vi "GetAllQueues.vi"(8 "error in (no error)":errorcluster, 11 "Qbus in":refnum<class "Qbus.lvclass">) -> (0 "error in (no error)":errorcluster, 2 "queues":refnum<queue>[](array[refnum]), 3 "Qbus out":refnum<class "Qbus.lvclass">)   [LabVIEW 2017, in "Qbus.lvclass"]
uses:
  <vilib>/addons/Qbus/Qbus.lvclass
  <vilib>/addons/Qbus/controls/message.ctl
  <vilib>/addons/Qbus/Qbus.lvclass/Qbus.ctl
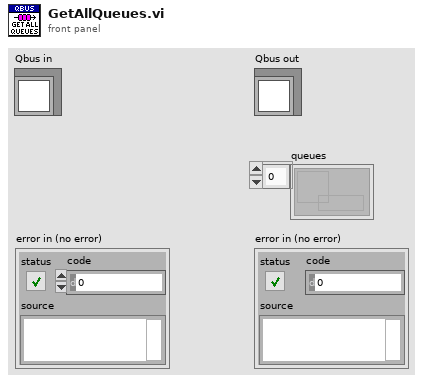
[diagram p1: front panel]
types:
  T1 = typedef "Qbus.lvclass/data.ctl" = cluster{"Queues":variant, "Subscriptions":variant, "MasterQ":string}
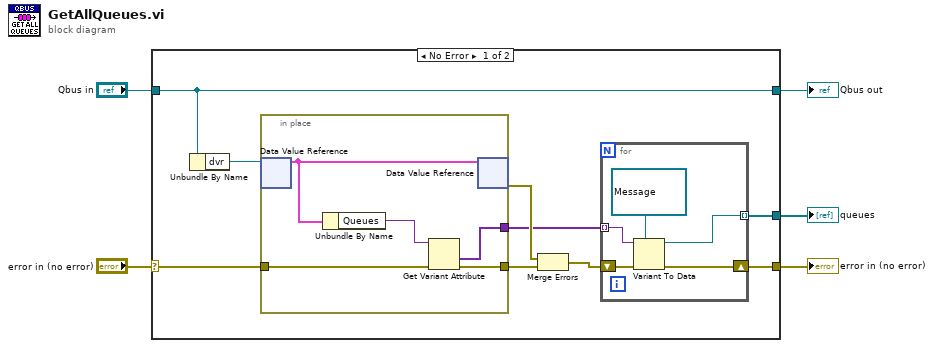
[diagram p0: block diagram]
diagram:
  n1 = case shown="No Error" "error in (no error)" {
    selector: "error in (no error)" -> [w11 w26]
    tunnel: [w8 w26] -> w4
    tunnel: [w14 w25] -> w2
    tunnel: "Qbus in" -> [w14 w25]
    tunnel: [w6 _] -> w1
    frame No Error {
      n2 = Unbundle By Name(w14) -> ("dvr"=w13:refnum<data-value>)
      n3 = in-place {
        in-place-border: w11 -> [w24]
        in-place-border: [w21] -> w10
        in-place-border: [w20] -> w7
        n4 = in-place-dvr #1(w13) -> (w22:T1)  [unwired: 1 out]
        n5 = Unbundle By Name(w22) -> ("Queues"=w23:variant)
        n6 = Get Variant Attribute(Variant=w23, error in=w24) -> (values=w20:variant[], error out=w21:errorcluster)  [unwired: 2 in, 2 out]
        n7 = in-place-dvr #1(w22) -> (w12:errorcluster)  [unwired: 1 out]
      }
      n8 = Merge Errors(w12, w10) -> (w9:errorcluster)
      n9 = for {
        shift-right: [w18] -> w8
        shift-left: w9 -> [w19]
        tunnel: w7 -> [w16] mode=indexing
        tunnel: [w15] -> w6 mode=indexing
        n10 = Variant To Data(error in=w19, type=refnum<queue> refnum ("queue out"), Variant=w16) -> (data=w15:refnum<queue>, error out=w18:errorcluster)
      }
    }
    frame Error {
    }
  }
  "error in (no error)" <- w4
  "Qbus out" <- w2
  "queues" <- w1
